vi "scripting_v1.vi"() -> ()   [LabVIEW 2020]
uses:
  <vilib>/numeric/LVNumericRepresentation.ctl
panel:
  out "error out 2":errorcluster
  in  "Target Name":string
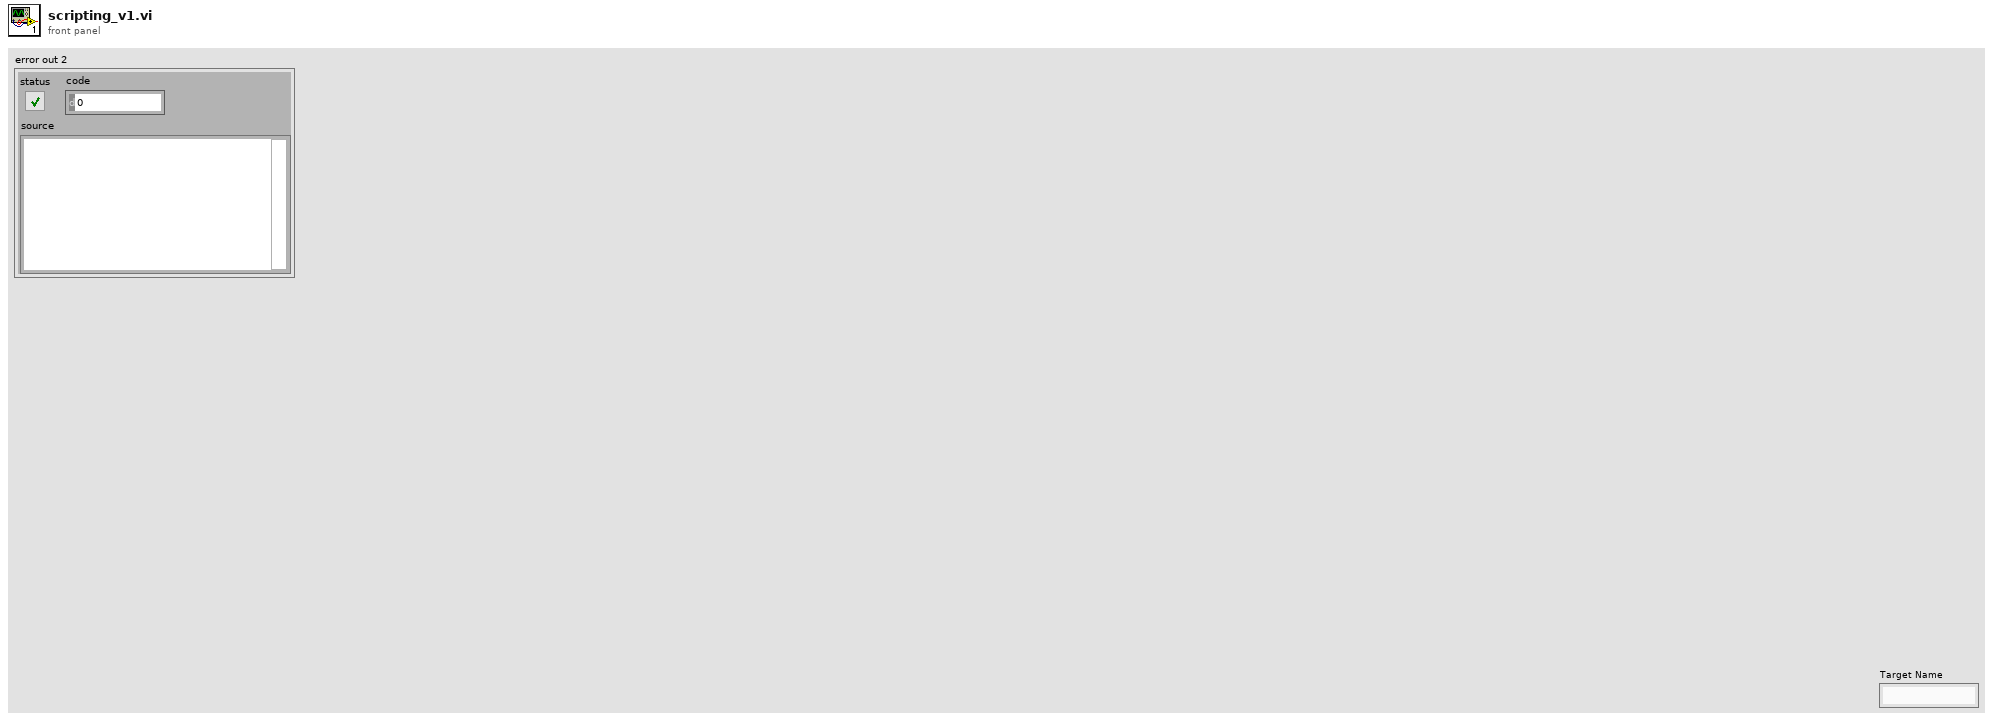
[diagram p1: front panel]
types:
  T1 = typedef "LVNumericRepresentation.ctl" = enum32{"Extended Precision", "Double Precision", "Single Precision", "Long", "Word", "Byte", "Unsigned Long", "Unsigned Word", "Unsigned Byte", "Complex Extended", "Complex Double", "Complex Single", "Quad", "Unsigned Quad", "Fixed-Point"}
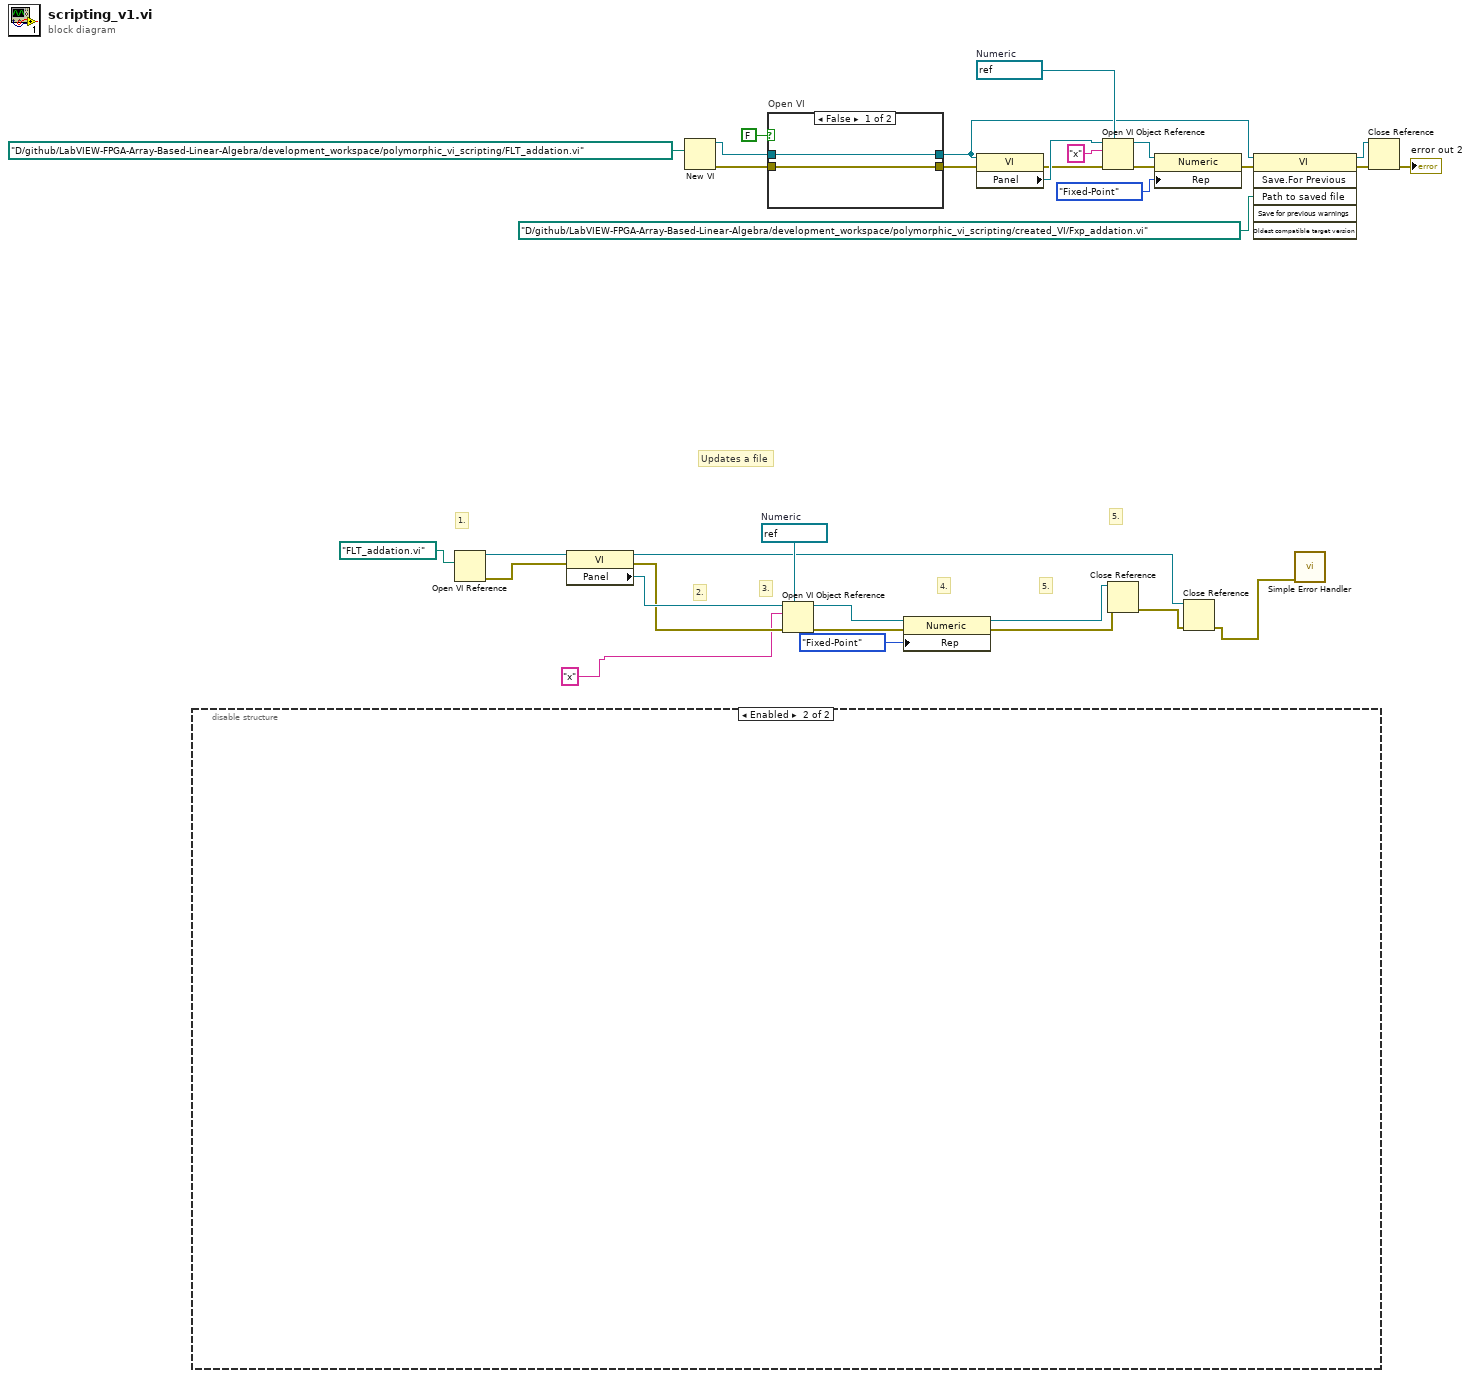
[diagram p0: block diagram]
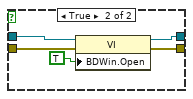
[diagram p2: hidden frame]
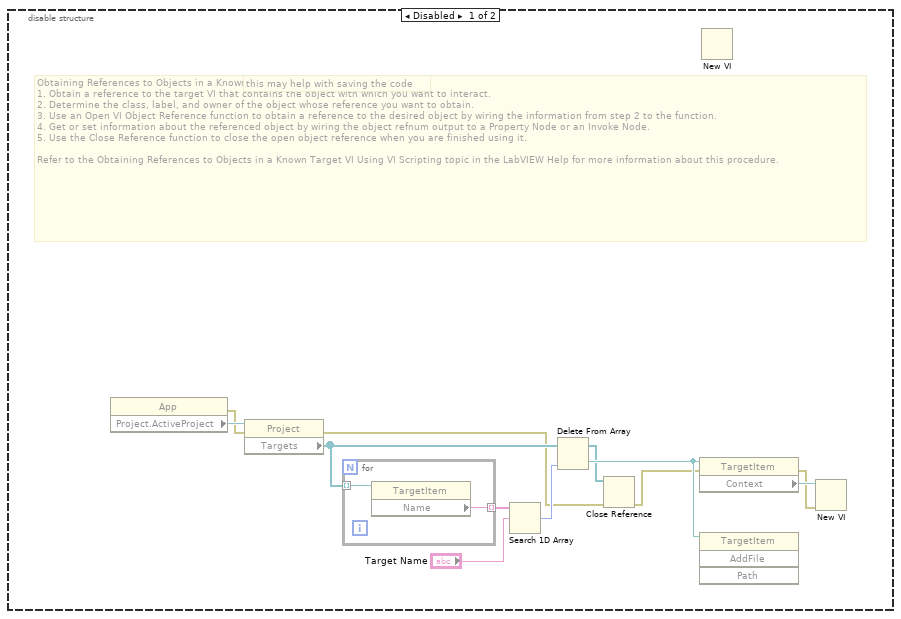
[diagram p3: hidden frame]
diagram:
  w10 = refnum<vi> refnum  # Numeric
  w33 = refnum<vi> refnum  # Numeric
  # "Updates a file"
  # "5."
  # "5."
  # "4."
  # "3."
  # "2."
  # "1."
  n1 = disable-structure shown="Enabled" {
    frame Disabled {
      # "this may help with saving the code"
      # "Obtaining References to Objects in a Known Target VI Using VI Scripting\n1. Obtain a reference to the target VI that contains the object with which you want to interact.\n2. Determine the class, label, and owner of the object whose reference you want to obtain.\n3. Use an Open VI Object Reference function to obtain a reference to the desired object by wiring the information from step 2 to the function.\n4. Get or set information about the referenced object by wiring the object refnum output to a Property Node or an Invoke Node.\n5. Use the Close Reference function to close the open object reference when you are finished using it.\n\nRefer to the Obtaining References to Objects in a Known Target VI Using VI Scripting topic in the LabVIEW Help for more information about this procedure."
      n2 = property class="App"() -> (error out=w34:errorcluster, "Project.ActiveProject"=w38:refnum<vi>)  [unwired: 2 in, 1 out]
      n3 = property class="Project"(reference=w38, error in=w34) -> (error out=w36:errorcluster, "Targets"=w41:refnum<vi>[])  [unwired: 1 out]
      n4 = for {
        tunnel: w41 -> [w47] mode=indexing
        tunnel: [w46] -> w39 mode=indexing
        n5 = property class="TargetItem"(reference=w47) -> ("Name"=w46:string)  [unwired: 1 in, 2 out]
      }
      n6 = Search 1D Array(1D array=w39, element="Target Name") -> (index of element=w42:i32)  [unwired: 1 in]
      n7 = Delete From Array(array=w41, index=w42) -> (deleted portion=w45:refnum<vi>, array with subset deleted=w43:refnum<vi>[])  [unwired: 1 in]
      n8 = Close Reference(reference=w43, error in (no error)=w36) -> (error out=w35:errorcluster)
      n9 = property class="TargetItem"(reference=w45, error in=w35) -> (error out=w37:errorcluster, "Context"=w44:refnum<vi>)  [unwired: 1 out]
      n10 = invoke class="TargetItem" method="AddFile"(reference=w45) -> ()  [unwired: 3 in, 4 out]
      n11 = New VI() -> ()  [unwired: 7 in, 2 out]
      n12 = New VI(8:w37, 11:w44) -> ()  [unwired: 5 in, 2 out]
    }
    frame Enabled {
    }
  }
  n13 = Open VI Reference(vi path=path "FLT_addation.vi") -> (vi reference=w26:refnum<vi>, error out=w27:errorcluster)  [unwired: 5 in]
  n14 = property on="Property Node" class="VI"(reference=w26, error in=w27) -> (reference out=w21:refnum<vi>, error out=w29:errorcluster, "Panel"=w31:refnum<vi>)
  n15 = New VI(10:path "D:/github/LabVIEW-FPGA-Array-Based-Linear-Algebra/development_workspace/polymorphic_vi_scripting/FLT_addation.vi" ("vi path")) -> (0:w17:errorcluster, 3:w18:refnum<vi>)  [unwired: 6 in]
  n16 = case "Open VI" shown="False" FALSE {
    tunnel: w18 -> [w48 w54]
    tunnel: w17 -> [w49 w53]
    tunnel: [w48 w51] -> w1
    tunnel: [w49 w50] -> w3
    frame False {
    }
    frame True {
      n17 = property class="VI"(reference=w54, error in=w53, "BDWin.Open"=TRUE ("Block Diagram Window:Open")) -> (reference out=w51:refnum<vi>, error out=w50:errorcluster)
    }
  }
  n18 = Open VI Object Reference(7:w33, 8:w29, 10:"x" ("name/order"), 11:w31) -> (0:w30:errorcluster, 3:w32:refnum<vi>)
  n19 = property on="Property Node" class="Numeric"(reference=w32, error in=w30, "Rep"=LVNumericRepresentation."Fixed-Point" ("new representation")) -> (reference out=w23:refnum<vi>, error out=w22:errorcluster)
  n20 = property on="Property Node" class="VI"(reference=w1, error in=w3) -> (error out=w6:errorcluster, "Panel"=w8:refnum<vi>)  [unwired: 1 out]
  n21 = Open VI Object Reference(7:w10, 8:w6, 10:"x" ("name/order"), 11:w8) -> (0:w7:errorcluster, 3:w9:refnum<vi>)
  n22 = Close Reference(reference=w23, error in (no error)=w22) -> (error out=w20:errorcluster)
  n23 = property on="Property Node" class="Numeric"(reference=w9, error in=w7, "Rep"=LVNumericRepresentation."Fixed-Point" ("new representation")) -> (error out=w2:errorcluster)  [unwired: 1 out]
  n24 = Close Reference(reference=w21, error in (no error)=w20) -> (error out=w19:errorcluster)
  n25 = invoke class="VI" method="Save.For Previous"(reference=w1, error in=w2, "Path to saved file"=path "D:/github/LabVIEW-FPGA-Array-Based-Linear-Algebra/development_workspace/polymorphic_vi_scripting/created_VI/Fxp_addation.vi" ("Path to Saved File")) -> (reference out=w16:refnum<vi>, error out=w15:errorcluster)  [unwired: 3 in, 4 out]
  n26 = call <vilib>:"Simple Error Handler.vi"("error in (no error)"=w19) -> ()  [unwired: 4 in, 5 out]
  n27 = Close Reference(reference=w16, error in (no error)=w15) -> (error out=→"error out 2":errorcluster)
